vi "Generate Create Thing JSON.vi"(10 "Thing Type JSON":string, 11 "Attributes":T1[](array[typedef])) -> (3 "Create Thing JSON":string)   [LabVIEW 2015, in "NI_AWS_IoT.lvlib"]
uses:
  NI_AWS_IoT.lvlib
  Core/HTTP Request/Name Value Pair.ctl
  Core/HTTP Request/HTTP Request.lvclass
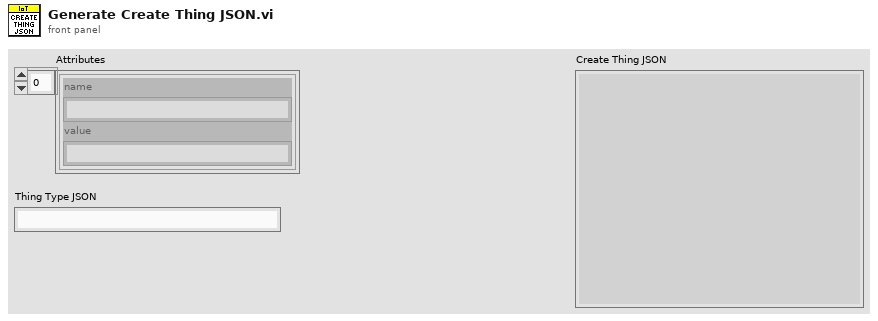
[diagram p1: front panel]
types:
  T1 = typedef "NI_AWS_Core.lvlib/HTTP Request.lvclass/Name Value Pair.ctl" = cluster{"name":string, "value":string}
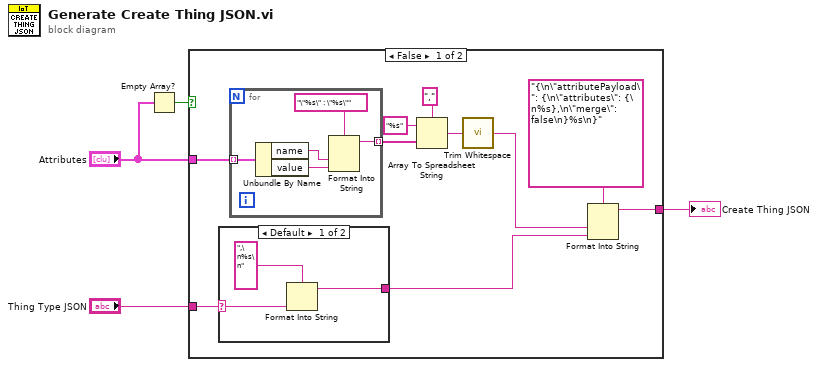
[diagram p0: block diagram]
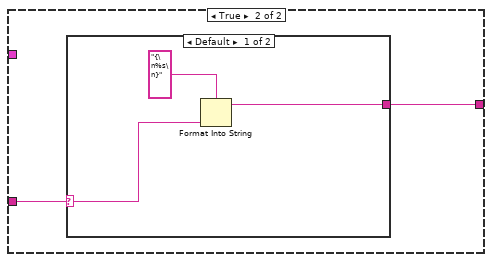
[diagram p3: hidden frame]
diagram:
  n1 = Empty Array?(array="Attributes") -> (empty?=w4:bool)
  n2 = case shown="False" w4 {
    tunnel: [w10 w23] -> w2
    tunnel: "Thing Type JSON" -> [w13 w24]
    tunnel: "Attributes" -> [w14 _]
    frame False {
      n3 = case shown="Default" w13 {
        selector: w13 -> [w17 _]
        tunnel: [w15 _] -> w11
        frame Default {
          n4 = Format Into String(format string=",\n%s\n", w17) -> (resulting string=w15:string)  [unwired: 2 in, 1 out]
        }
        frame "" {
        }
      }
      n5 = for {
        tunnel: w14 -> [w22] mode=indexing
        tunnel: [w18] -> w9 mode=indexing
        n6 = Unbundle By Name(w22) -> ("name"=w19:string, "value"=w20:string)
        n7 = Format Into String(format string="\"%s\" : \"%s\"", w19, w20) -> (resulting string=w18:string)  [unwired: 2 in, 1 out]
      }
      n8 = Array To Spreadsheet String(delimiter (Tab)=",", array=w9, 3:"%s" ("format string")) -> (spreadsheet string=w8:string)
      n9 = call <vilib>:"Trim Whitespace.vi"("string"=w8) -> ("trimmed string"=w6:string)  [unwired: 1 in]
      n10 = Format Into String(format string="{\n\"attributePayload\": {\n\"attributes\": {\n%s},\n\"merge\": false\n}%s\n}", w6, w11) -> (resulting string=w10:string)  [unwired: 2 in, 1 out]
    }
    frame True {
      n11 = case shown="Default" w24 {
        selector: w24 -> [w26 _]
        tunnel: [w25 _] -> w23
        frame Default {
          n12 = Format Into String(format string="{\n%s\n}", w26) -> (resulting string=w25:string)  [unwired: 2 in, 1 out]
        }
        frame "" {
        }
      }
    }
  }
  "Create Thing JSON" <- w2
